vi "Example2.2-ShiftRegisterb.vi"() -> ()   [LabVIEW 2019]
panel:
  out "Time Between Loop Iterations":dbl
  in  "ms to Wait":dbl=50.0
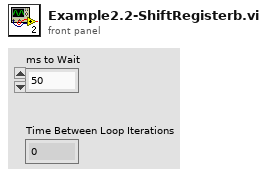
[diagram p1: front panel]
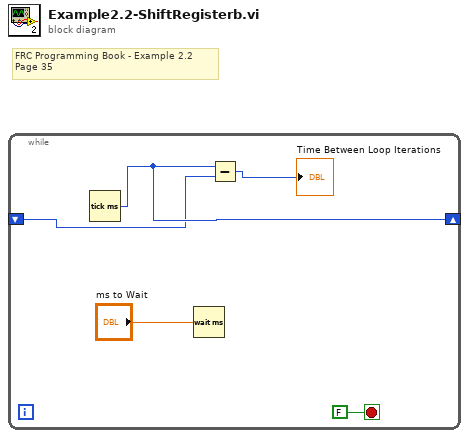
[diagram p0: block diagram]
diagram:
  # "FRC Programming Book - Example 2.2\nPage 35"
  n1 = while {
    shift-right: [w4] -> _
    shift-left: _ -> [w3]
    stop <- FALSE stop-if-true
    n2 = Tick Count (ms)() -> (millisecond timer value=w4:u32)
    n3 = Wait (ms)(milliseconds to wait="ms to Wait") -> ()  [unwired: 1 out]
    n4 = Subtract(x=w4, y=w3) -> (x-y=→"Time Between Loop Iterations":u32)
  }
